vi "Close vi references.vi"(11 "map":map{string, refnum<vi>}(c390)) -> (0 "error out":errorcluster)   [LabVIEW 2020, in "Panter Dashboard.lvlib"]
uses:
  Panter Dashboard.lvlib
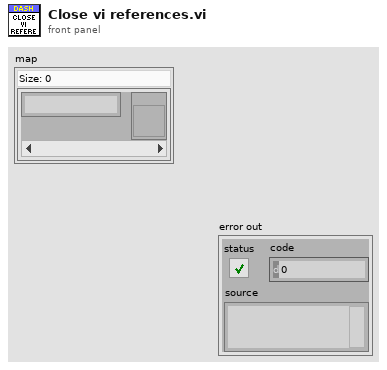
[diagram p1: front panel]
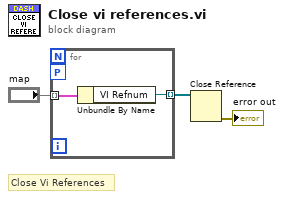
[diagram p0: block diagram]
diagram:
  # "Close Vi References"
  n1 = for {
    tunnel: "map" -> [w5] mode=indexing
    tunnel: [w4] -> w3 mode=indexing
    workers-P: _ -> [_]
    n2 = Unbundle By Name(w5) -> ("VI Refnum"=w4:refnum<vi>)
  }
  n3 = Close Reference(reference=w3) -> (error out=→"error out":errorcluster)  [unwired: 1 in]
